vi "NIIE_MouseMove.vi"(7 "Buffer":refnum<queue>, 8 "Error":errorcluster, 9 "Coords":T5, 11 "Data":T1={"Class"={"Ants"=refnum, "Layer"=refnum, "Templates"=refnum, "Icon"=refnum, "Glyph"=refnum, "Settings"=refnum, "Tools"=refnum}, "Ref"={"Add Layer"=refnum, "Remove Layer"=refnum, "Line Text"=[], "Body Text Spec"=refnum, "DNL_Font"=refnum, "glyph path str"=refnum, "templates path str"=refnum, "Arrow Up"=refnum, "Arrow Down"=refnum, "IE VI Ref"=refnum, "Glyphs tree"=refnum, "Templates tree"=refnum, "Layer Icon Text"=refnum, "Layer Template"=refnum, "Clipboard"=refnum, "BW icon in"=refnum, "Color icon in"=refnum, "Layer Clust"=refnum, "Body Text"=refnum, "DNL_Framework Templates"=refnum, "Search Templates"=refnum, "TextMarker"=refnum, "Tab Control"=refnum, "Search Glyphs"=refnum, "Line Color"=refnum, "DNL_Glyphs []"=refnum, "Fill Color"=refnum, "Tools"=refnum, "Glyphs tree"=refnum, "Icon"=refnum, "Preview"=refnum, "Ants"=refnum, "Terminals"=refnum, "menu reference"=refnum, "LayerNames"=[], "GlyphLoadAnimation"=refnum, "TemplateLoadAnimation"=refnum, "refreshGlyphs"=refnum, "refreshTemplates"=refnum}, "Support"={"AntsRect"={"left"=0, "top"=0, "right"=0, "bottom"=0}, "Mouse Move Coords"={"Horizontal"=0, "Vertical"=0}, "Mouse Down Coords"={"Horizontal"=0, "Vertical"=0}, "Temp Coord"={"Horizontal"=0, "Vertical"=0}, "Action"=enum."Default", "Edge Color"=4914962, "Fill Color"=16860, "Mouse Down?"=FALSE, "Draft Mode?"=FALSE, "Temp Icon"=bytes[3102], "CTRL Pressed"=FALSE, "Move Selection?"=FALSE, "AntsRect Orig"={"left"=0, "top"=0, "right"=0, "bottom"=0}, "Text"="", "TM Set?"=FALSE, "Mouse inside icon?"=FALSE, "Tool (old value)"=0, "Pencil Move Color"=0, "Swap Colors?"=FALSE, "Shift pressed?"=FALSE}}) -> (0 "Error Out":errorcluster, 3 "Data Out":T1={"Class"={"Ants"=refnum, "Layer"=refnum, "Templates"=refnum, "Icon"=refnum, "Glyph"=refnum, "Settings"=refnum, "Tools"=refnum}, "Ref"={"Add Layer"=refnum, "Remove Layer"=refnum, "Line Text"=[], "Body Text Spec"=refnum, "DNL_Font"=refnum, "glyph path str"=refnum, "templates path str"=refnum, "Arrow Up"=refnum, "Arrow Down"=refnum, "IE VI Ref"=refnum, "Glyphs tree"=refnum, "Templates tree"=refnum, "Layer Icon Text"=refnum, "Layer Template"=refnum, "Clipboard"=refnum, "BW icon in"=refnum, "Color icon in"=refnum, "Layer Clust"=refnum, "Body Text"=refnum, "DNL_Framework Templates"=refnum, "Search Templates"=refnum, "TextMarker"=refnum, "Tab Control"=refnum, "Search Glyphs"=refnum, "Line Color"=refnum, "DNL_Glyphs []"=refnum, "Fill Color"=refnum, "Tools"=refnum, "Glyphs tree"=refnum, "Icon"=refnum, "Preview"=refnum, "Ants"=refnum, "Terminals"=refnum, "menu reference"=refnum, "LayerNames"=[], "GlyphLoadAnimation"=refnum, "TemplateLoadAnimation"=refnum, "refreshGlyphs"=refnum, "refreshTemplates"=refnum}, "Support"={"AntsRect"={"left"=0, "top"=0, "right"=0, "bottom"=0}, "Mouse Move Coords"={"Horizontal"=0, "Vertical"=0}, "Mouse Down Coords"={"Horizontal"=0, "Vertical"=0}, "Temp Coord"={"Horizontal"=0, "Vertical"=0}, "Action"=enum."Default", "Edge Color"=4914962, "Fill Color"=16860, "Mouse Down?"=FALSE, "Draft Mode?"=FALSE, "Temp Icon"=bytes[3102], "CTRL Pressed"=FALSE, "Move Selection?"=FALSE, "AntsRect Orig"={"left"=0, "top"=0, "right"=0, "bottom"=0}, "Text"="", "TM Set?"=FALSE, "Mouse inside icon?"=FALSE, "Tool (old value)"=0, "Pencil Move Color"=0, "Swap Colors?"=FALSE, "Shift pressed?"=FALSE}})   [LabVIEW 2021]
uses:
  <vilib>/Utility/miscctls.llb/LVPoint32TypeDef.ctl
  Controls/IE Data.ctl
  Class/Ants/Ants.lvclass
  Class/FakedArray/FakedArray.lvclass
  Class/Icon Library/Glyph.lvclass
  Class/Settings/Settings.lvclass
  Class/Tools/Tools Paint.lvclass
  vi.lib/LabVIEW Icon API/lv_icon/Classes/Icon/Icon.lvclass
  Controls/IE Classes.ctl
  Controls/References Cluster.ctl
  Controls/SupportClass.ctl
  Controls/ENUM_SupportClass_Action.ctl
  vi.lib/LabVIEW Icon API/lv_icon/Controls/IEColor.ctl
  vi.lib/LabVIEW Icon API/lv_icon/lv_icon.lvlib
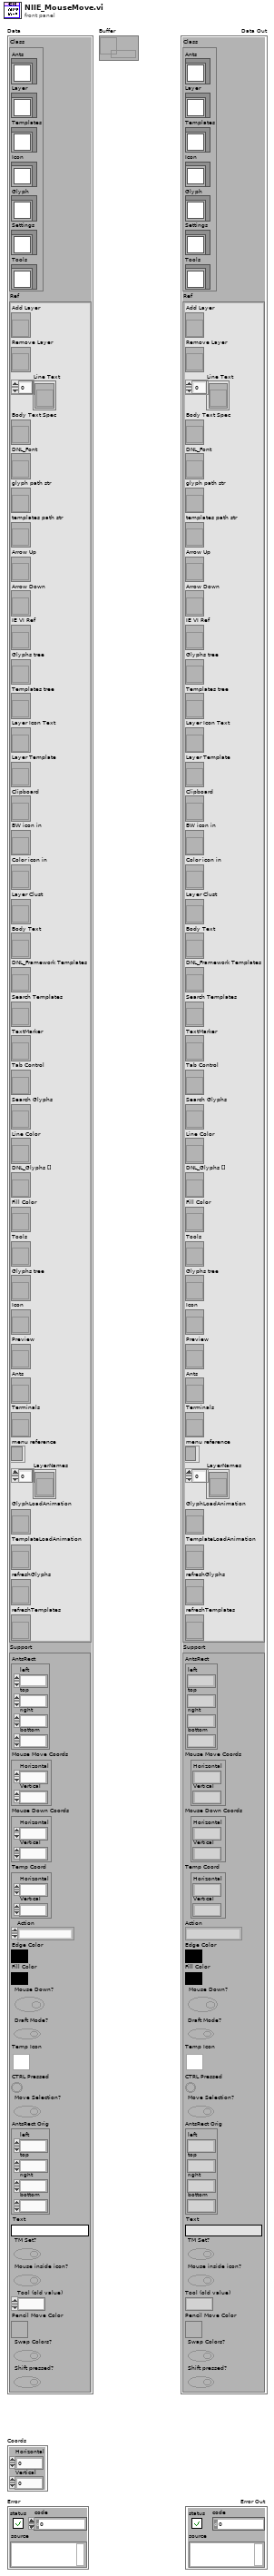
[diagram p1: front panel]
types:
  T1 = typedef "IE Data.ctl" = cluster{"Class":T2, "Ref":T3, "Support":T4}
  T2 = typedef "IE Classes.ctl" = cluster{"Ants":refnum<class "Ants.lvclass">, "Layer":refnum<class "FakedArray.lvclass">, "Templates":refnum<class "FakedArray.lvclass">, "Icon":refnum<class "Icon.lvclass">, "Glyph":refnum<class "Glyph.lvclass">, "Settings":refnum<class "Settings.lvclass">, "Tools":refnum<class "Tools Paint.lvclass">}
  T3 = typedef "References Cluster.ctl" = cluster{"Add Layer":refnum<vi>, "Remove Layer":refnum<vi>, "Line Text":refnum<vi>[], "Body Text Spec":refnum<vi>, "DNL_Font":refnum<vi>, "glyph path str":refnum<vi>, "templates path str":refnum<vi>, "Arrow Up":refnum<vi>, "Arrow Down":refnum<vi>, "IE VI Ref":refnum<vi>, "Glyphs tree":refnum<vi>, "Templates tree":refnum<vi>, "Layer Icon Text":refnum<vi>, "Layer Template":refnum<vi>, "Clipboard":refnum<vi>, "BW icon in":refnum<vi>, "Color icon in":refnum<vi>, "Layer Clust":refnum<vi>, "Body Text":refnum<vi>, "DNL_Framework Templates":refnum<vi>, "Search Templates":refnum<vi>, "TextMarker":refnum<vi>, "Tab Control":refnum<vi>, "Search Glyphs":refnum<vi>, "Line Color":refnum<vi>, "DNL_Glyphs []":refnum<vi>, "Fill Color":refnum<vi>, "Tools":refnum<vi>, "Glyphs tree":refnum<vi>, "Icon":refnum<vi>, "Preview":refnum<vi>, "Ants":refnum<vi>, "Terminals":refnum<vi>, "menu reference":refnum<k9>, "LayerNames":refnum<vi>[], "GlyphLoadAnimation":refnum<vi>, "TemplateLoadAnimation":refnum<vi>, "refreshGlyphs":refnum<vi>, "refreshTemplates":refnum<vi>}
  T4 = typedef "SupportClass.ctl" = cluster{"AntsRect":cluster{"left":i16, "top":i16, "right":i16, "bottom":i16}, "Mouse Move Coords":T5, "Mouse Down Coords":T5, "Temp Coord":T5, "Action":T6, "Edge Color":T7, "Fill Color":T7, "Mouse Down?":bool, "Draft Mode?":bool, "Temp Icon":picture, "CTRL Pressed":bool, "Move Selection?":bool, "AntsRect Orig":cluster{"left":i16, "top":i16, "right":i16, "bottom":i16}, "Text":string, "TM Set?":bool, "Mouse inside icon?":bool, "Tool (old value)":u32, "Pencil Move Color":u32, "Swap Colors?":bool, "Shift pressed?":bool}
  T5 = typedef "LVPoint32TypeDef.ctl" = cluster{"Horizontal":i32, "Vertical":i32}
  T6 = typedef "ENUM_SupportClass_Action.ctl" = enum16{"Default", "Move Selection", "Glyph Library", "Tool"}
  T7 = typedef "IEColor.ctl" = u32
  T8 = typedef "Cluster_Path&Icon.ctl" = cluster{"Rectangle":cluster{"left":i16, "top":i16, "right":i16, "bottom":i16}, "Path":path, "Image":picture, "Filter":string, "FileName":string}
  T9 = cluster{"left":i16, "top":i16, "right":i16, "bottom":i16}
  T10 = typedef "Cluster_Button Draw Tools.ctl" = enum32{"Pencil", "Line", "Dropper", "Fill", "Rectangle", "Filled Rectangle", "Ellipse", "Filled Ellipse", "Eraser", "Text", "Select", "Move"}
  T11 = cluster{"Horizontal":i32, "Vertical":i32, "Horizontal":i32, "Vertical":i32}
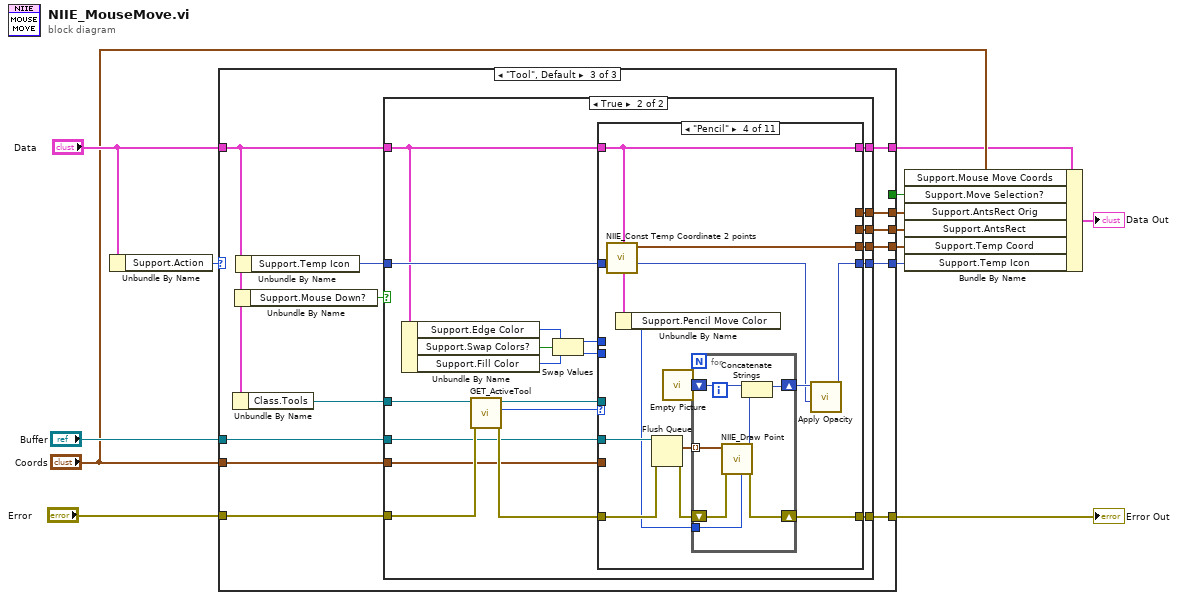
[diagram p0: block diagram]
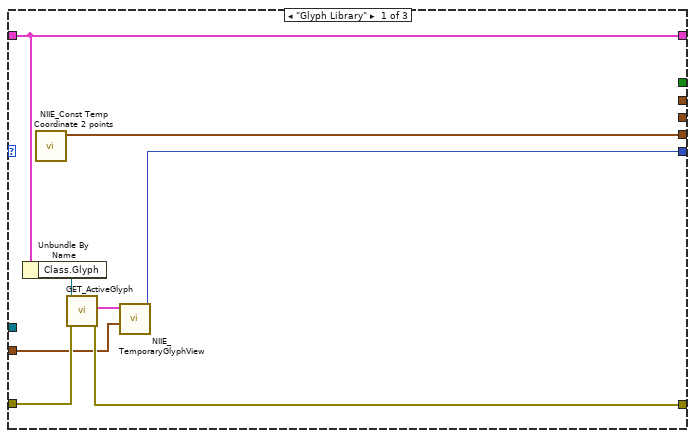
[diagram p2: hidden frame]
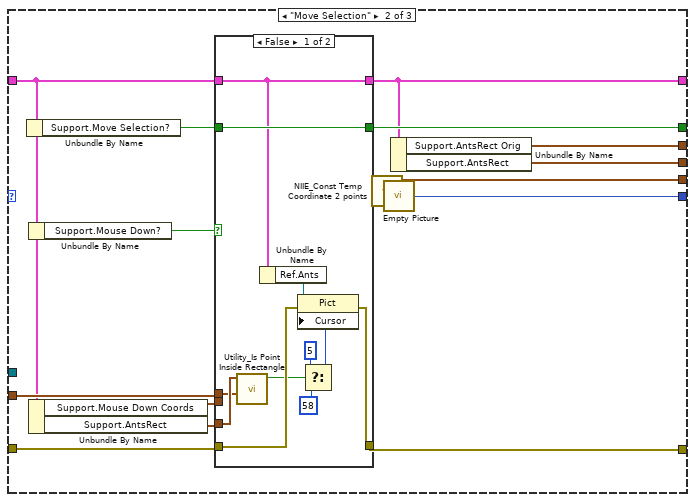
[diagram p3: hidden frame]
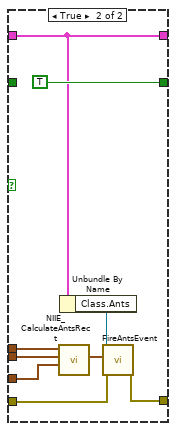
[diagram p4: hidden frame]
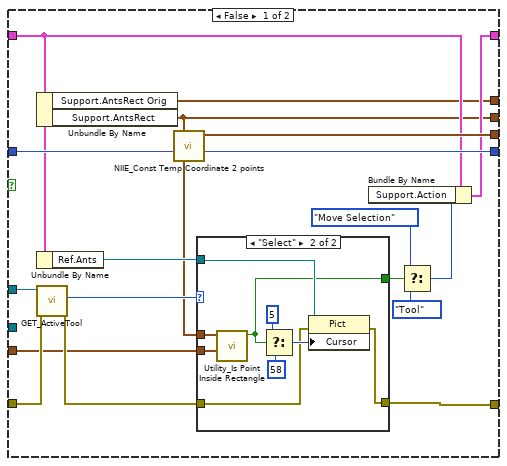
[diagram p5: hidden frame]
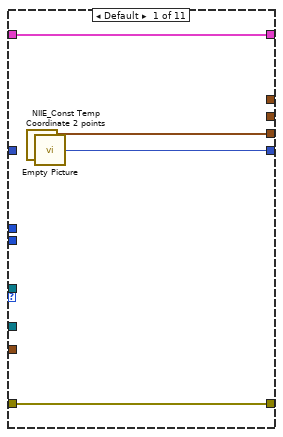
[diagram p7: hidden frame]
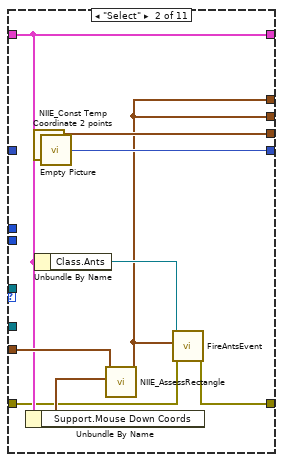
[diagram p8: hidden frame]
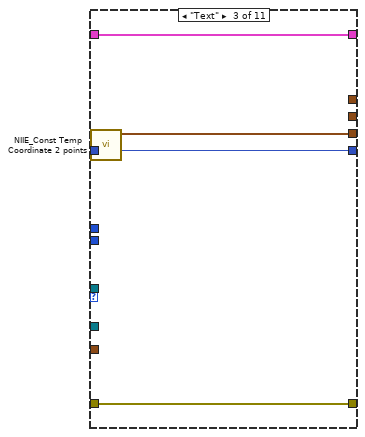
[diagram p9: hidden frame]
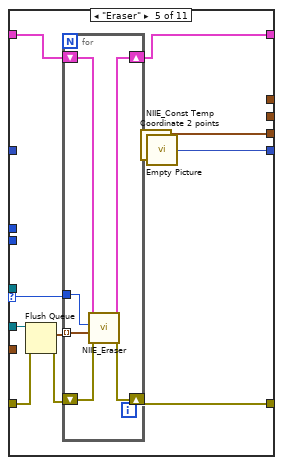
[diagram p10: hidden frame]
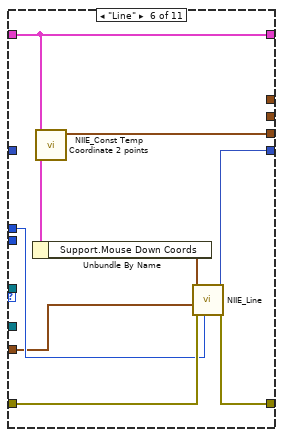
[diagram p11: hidden frame]
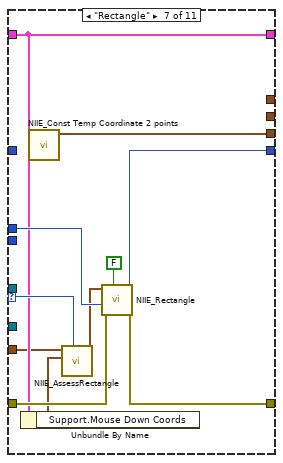
[diagram p12: hidden frame]
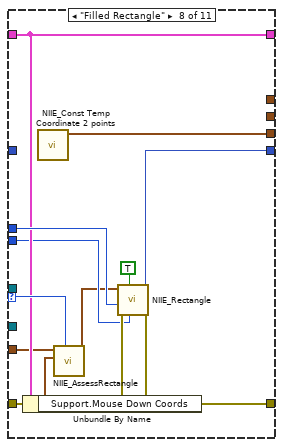
[diagram p13: hidden frame]
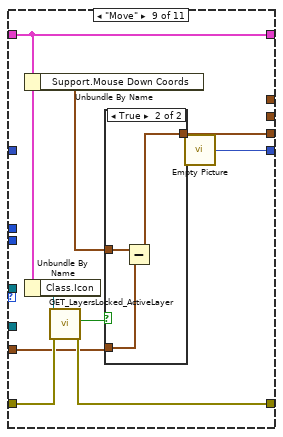
[diagram p14: hidden frame]
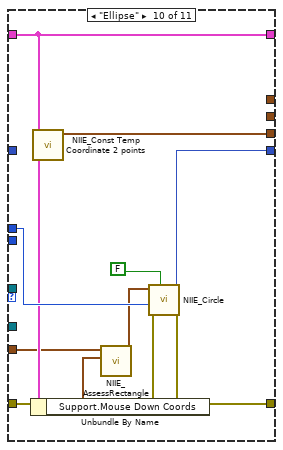
[diagram p16: hidden frame]
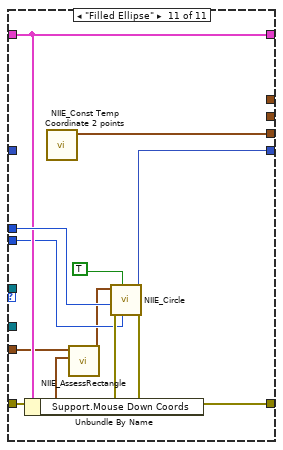
[diagram p17: hidden frame]
diagram:
  n1 = Unbundle By Name("Data") -> ("Support.Action"=w11:T6)
  n2 = case shown="\"Tool\", Default" w11 {
    tunnel: "Error" -> [w17 w33 w68]
    tunnel: [w20 w32 w67] -> w5
    tunnel: [w19 w34 w66] -> w12
    tunnel: [w18 w35 w65] -> w13
    tunnel: [_ w28 w64] -> w10
    tunnel: [_ w29 w63] -> w9
    tunnel: [_ w31 _] -> w8
    tunnel: "Buffer" -> [_ _ w62]
    tunnel: "Data" -> [w15 w23 w57]
    tunnel: [w15 w22 w61] -> w1
    tunnel: "Coords" -> [w14 w30 w60]
    frame "Glyph Library" {
      n3 = Unbundle By Name(w15) -> ("Class.Glyph"=w16:refnum<class "Glyph.lvclass">)
      n4 = call "NIIE_Const Temp Coordinate 2 points.vi"() -> ("Const Temp Coordinate"=w18:T5)  [unwired: 11 out]
      n5 = call-dynamic "GET_ActiveGlyph.vi"("Error"=w17, "Glyph.lvclass"=w16) -> ("Error Out"=w20:errorcluster, "Path And Icon Out"=w21:T8)  [unwired: 8 out]
      n6 = call "NIIE_TemporaryGlyphView.vi"("Mouse Coords Pic"=w14, "Path And Icon"=w21) -> ("Icon Out"=w19:picture)  [unwired: 9 out]
    }
    frame "Move Selection" {
      n7 = Unbundle By Name(w23) -> ("Support.Move Selection?"=w24:bool)
      n8 = Unbundle By Name(w23) -> ("Support.Mouse Down?"=w25:bool)
      n9 = Unbundle By Name(w23) -> ("Support.Mouse Down Coords"=w26:T5, "Support.AntsRect"=w27:T9)
      n10 = case shown="False" w25 {
        tunnel: w33 -> [w39 w55]
        tunnel: [w43 w54] -> w32
        tunnel: w30 -> [w40 w49]
        tunnel: w26 -> [_ w52]
        tunnel: w27 -> [w42 w51]
        tunnel: [w41 TRUE] -> w31
        tunnel: w24 -> [w41 _]
        tunnel: w23 -> [w37 w47]
        tunnel: [w37 w47] -> w22
        frame False {
          n11 = call "Utility_Is Point Inside Rectangle.vi"("Point"=w40, "Rectangle"=w42) -> ("Inside? Out"=w36:bool)  [unwired: 9 out]
          n12 = Unbundle By Name(w37) -> ("Ref.Ants"=w38:refnum<vi>)
          n13 = Select(t=5 ("Cursor"), s=w36, f=58 ("Cursor")) -> (s? t:f=w44:i32)
          n14 = property class="Pict"(reference=w38, error in=w39, "Cursor"=w44) -> (error out=w43:errorcluster)  [unwired: 1 out]
        }
        frame True {
          n15 = call "NIIE_CalculateAntsRect.vi"("AntsRect"=w51, "Mouse Down Coords"=w52, "Mouse Move Coords"=w49) -> ("Rect"=w50:cluster{i32, i32, i32, i32})  [unwired: 8 out]
          n16 = Unbundle By Name(w47) -> ("Class.Ants"=w48:refnum<class "Ants.lvclass">)
          n17 = call "FireAntsEvent.vi"("error in (no error)"=w55, "Rectangle (default: deselect)"=w50, "Ants in"=w48) -> ("error out"=w54:errorcluster)  [unwired: 1 in, 7 out]
        }
      }
      n18 = call "NIIE_Const Temp Coordinate 2 points.vi"() -> ("Const Temp Coordinate"=w35:T5)  [unwired: 11 out]
      n19 = call "Empty Picture"() -> ("empty picture"=w34:picture)
      n20 = Unbundle By Name(w22) -> ("Support.AntsRect Orig"=w29:T9, "Support.AntsRect"=w28:T9)
    }
    frame "Tool", Default {
      n21 = Unbundle By Name(w57) -> ("Class.Tools"=w59:refnum<class "Tools Paint.lvclass">)
      n22 = Unbundle By Name(w57) -> ("Support.Mouse Down?"=w58:bool)
      n23 = Unbundle By Name(w57) -> ("Support.Temp Icon"=w56:picture)
      n24 = case shown="True" w58 {
        tunnel: w68 -> [w78 w115]
        tunnel: w56 -> [w77 w112]
        tunnel: [w82 w110] -> w67
        tunnel: [w77 w109] -> w66
        tunnel: [w85 w108] -> w65
        tunnel: [w70 w107] -> w64
        tunnel: [w69 w106] -> w63
        tunnel: w59 -> [w79 w105]
        tunnel: w62 -> [_ w104]
        tunnel: w57 -> [w72 w98]
        tunnel: [w76 w103] -> w61
        tunnel: w60 -> [w73 w102]
        frame False {
          n25 = Unbundle By Name(w72) -> ("Support.AntsRect Orig"=w69:T9, "Support.AntsRect"=w70:T9)
          n26 = Unbundle By Name(w72) -> ("Ref.Ants"=w74:refnum<vi>)
          n27 = call-dynamic "GET_ActiveTool.vi"("error in (no error)"=w78, "Tools Paint.lvclass in"=w79) -> ("error out"=w84:errorcluster, "Radio Buttons"=w83:T10)  [unwired: 8 out]
          n28 = call "NIIE_Const Temp Coordinate 2 points.vi"() -> ("Const Temp Coordinate"=w85:T5)  [unwired: 11 out]
          n29 = case shown="\"Select\"" w83 {
            tunnel: w84 -> [w86 w89]
            tunnel: w73 -> [_ w92]
            tunnel: [w86 w91] -> w82
            tunnel: w70 -> [_ w90]
            tunnel: [_ w87] -> w81
            tunnel: w74 -> [_ w88]
            frame Default {
            }
            frame "Select" {
              n30 = call "Utility_Is Point Inside Rectangle.vi"("Point"=w92, "Rectangle"=w90) -> ("Inside? Out"=w87:bool)  [unwired: 9 out]
              n31 = Select(t=5 ("Cursor"), s=w87, f=58 ("Cursor")) -> (s? t:f=w93:i32)
              n32 = property class="Pict"(reference=w88, error in=w89, "Cursor"=w93) -> (error out=w91:errorcluster)  [unwired: 1 out]
            }
          }
          n33 = Select(t=ENUM_SupportClass_Action."Move Selection", s=w81, f=ENUM_SupportClass_Action."Tool" ("t")) -> (s? t:f=w75:T6)
          n34 = Bundle By Name(cluster=w72, "Support.Action"=w75) -> (w76:T1)
        }
        frame True {
          n35 = Unbundle By Name(w98) -> ("Support.Edge Color"=w100:T7, "Support.Swap Colors?"=w101:bool, "Support.Fill Color"=w99:T7)
          n36 = call-dynamic "GET_ActiveTool.vi"("error in (no error)"=w115, "Tools Paint.lvclass in"=w105) -> ("error out"=w113:errorcluster, "Radio Buttons"=w114:T10, "Tools Paint.lvclass out"=w111:refnum<class "Tools Paint.lvclass">)  [unwired: 7 out]
          n37 = Swap Values(12:w100, 13:w101, 14:w99) -> (1:w96:T7, 3:w97:T7)
          n38 = case shown="\"Pencil\"" w114 {
            selector: w114 -> [_ _ _ _ w159 _ w183 w195 _ _ _]
            tunnel: w113 -> [w119 w120 w132 w136 w154 w175 w186 w198 w204 w220 w231]
            tunnel: w112 -> [_ _ w131 w137 _ _ _ _ _ _ _]
            tunnel: w111 -> [_ _ _ _ _ _ _ _ _ _ _]
            tunnel: w96 -> [_ _ _ _ _ w173 w184 w196 _ w218 w229]
            tunnel: [w119 w121 w132 w144 w161 w174 w185 w197 w206 w219 w230] -> w110
            tunnel: [w118 w127 w131 w143 w160 w168 w176 w187 w207 w212 w222] -> w109
            tunnel: [w117 w128 w130 w142 w158 w172 w182 w194 w201 w217 w228] -> w108
            tunnel: [_ w122 _ _ _ _ _ _ _ _ _] -> w107
            tunnel: [_ w122 _ _ _ _ _ _ _ _ _] -> w106
            tunnel: w97 -> [_ _ _ _ _ _ _ w191 _ _ w224]
            tunnel: w104 -> [_ _ _ w141 w155 _ _ _ _ _ _]
            tunnel: w98 -> [w116 w124 w129 w134 w157 w171 w181 w193 w200 w215 w226]
            tunnel: [w116 w124 w129 w134 w156 w171 w181 w193 w200 w215 w226] -> w103
            tunnel: w102 -> [_ w125 _ _ _ w170 w178 w189 w199 w213 w223]
            frame Default {
              n39 = call "NIIE_Const Temp Coordinate 2 points.vi"() -> ("Const Temp Coordinate"=w117:T5)  [unwired: 11 out]
              n40 = call "Empty Picture"() -> ("empty picture"=w118:picture)
            }
            frame "Select" {
              n41 = Unbundle By Name(w124) -> ("Support.Mouse Down Coords"=w126:T5)
              n42 = call "NIIE_Const Temp Coordinate 2 points.vi"() -> ("Const Temp Coordinate"=w128:T5)  [unwired: 11 out]
              n43 = Unbundle By Name(w124) -> ("Class.Ants"=w123:refnum<class "Ants.lvclass">)
              n44 = call "Empty Picture"() -> ("empty picture"=w127:picture)
              n45 = call "NIIE_AssessRectangle.vi"(10:"Coords"=w126, 11:"Coords"=w125) -> ("Rectangle Out"=w122:T11)  [unwired: 9 in]
              n46 = call "FireAntsEvent.vi"("error in (no error)"=w120, "Rectangle (default: deselect)"=w122, "Ants in"=w123) -> ("error out"=w121:errorcluster)  [unwired: 1 in, 7 out]
            }
            frame "Text" {
              n47 = call "NIIE_Const Temp Coordinate 2 points.vi"() -> ("Const Temp Coordinate"=w130:T5)  [unwired: 11 out]
            }
            frame "Pencil" {
              n48 = call "NIIE_Const Temp Coordinate 2 points.vi"() -> ("Const Temp Coordinate"=w142:T5)  [unwired: 11 out]
              n49 = Unbundle By Name(w134) -> ("Support.Pencil Move Color"=w133:u32)
              n50 = Flush Queue(queue=w141, error in (no error)=w136) -> (remaining elements=w135:T5[], error out=w140:errorcluster)  [unwired: 1 out]
              n51 = call "Empty Picture"() -> ("empty picture"=w139:picture)
              n52 = for {
                shift-right: [w151] -> w144
                shift-left: w140 -> [w150]
                tunnel: w135 -> [w145] mode=indexing
                shift-right: [w148] -> w138
                shift-left: w139 -> [w149]
                tunnel: w133 -> [w147]
                n53 = call "NIIE_Draw Point.vi"("Edge Color"=w147, "Error"=w150, "Point(x,y)"=w145) -> ("Error Out"=w151:errorcluster, "New Picture Out"=w146:picture)  [unwired: 6 in, 1 out]
                n54 = Concatenate Strings(w149, w146) -> (w148:picture)
              }
              n55 = call "Apply Opacity.vi"("Bottom"=w137, "Top"=w138) -> ("new picture"=w143:picture)  [unwired: 1 in, 8 out]
            }
            frame "Eraser" {
              n56 = Flush Queue(queue=w155, error in (no error)=w154) -> (remaining elements=w152:T5[], error out=w153:errorcluster)  [unwired: 1 out]
              n57 = for {
                tunnel: w159 -> [w165]
                shift-right: [w163] -> w156
                shift-left: w157 -> [w164]
                tunnel: w152 -> [w162] mode=indexing
                shift-right: [w167] -> w161
                shift-left: w153 -> [w166]
                n58 = call "NIIE_Eraser.vi"("Error"=w166, "Point Out"=w162, "Radio Buttons"=w165, "Data"=w164) -> ("Error Out"=w167:errorcluster, "Data Out"=w163:T1)  [unwired: 6 out]
              }
              n59 = call "NIIE_Const Temp Coordinate 2 points.vi"() -> ("Const Temp Coordinate"=w158:T5)  [unwired: 11 out]
              n60 = call "Empty Picture"() -> ("empty picture"=w160:picture)
            }
            frame "Line" {
              n61 = Unbundle By Name(w171) -> ("Support.Mouse Down Coords"=w169:T5)
              n62 = call "NIIE_Const Temp Coordinate 2 points.vi"() -> ("Const Temp Coordinate"=w172:T5)  [unwired: 11 out]
              n63 = call "NIIE_Line.vi"("Color(black)"=w173, "Error"=w175, "End Point"=w170, "New Position"=w169) -> ("Error Out"=w174:errorcluster, "New Picture Out"=w168:picture)  [unwired: 6 in]
            }
            frame "Rectangle" {
              n64 = Unbundle By Name(w181) -> ("Support.Mouse Down Coords"=w180:T5)
              n65 = call "NIIE_Const Temp Coordinate 2 points.vi"() -> ("Const Temp Coordinate"=w182:T5)  [unwired: 11 out]
              n66 = call "NIIE_AssessRectangle.vi"("Tool"=w183, 10:"Coords"=w180, 11:"Coords"=w178) -> ("Rectangle Out"=w177:T11)  [unwired: 8 in]
              n67 = call "NIIE_Rectangle.vi"("Fill?(F)"=FALSE, "Error"=w186, "Edge Color"=w184, "Rect"=w177) -> ("Error Out"=w185:errorcluster, "New Picture Out"=w176:picture)  [unwired: 6 in]
            }
            frame "Filled Rectangle" {
              n68 = Unbundle By Name(w193) -> ("Support.Mouse Down Coords"=w192:T5)
              n69 = call "NIIE_Const Temp Coordinate 2 points.vi"() -> ("Const Temp Coordinate"=w194:T5)  [unwired: 11 out]
              n70 = call "NIIE_AssessRectangle.vi"("Tool"=w195, 10:"Coords"=w192, 11:"Coords"=w189) -> ("Rectangle Out"=w188:T11)  [unwired: 8 in]
              n71 = call "NIIE_Rectangle.vi"("Fill Color"=w191, "Fill?(F)"=TRUE, "Error"=w198, "Edge Color"=w196, "Rect"=w188) -> ("Error Out"=w197:errorcluster, "New Picture Out"=w187:picture)  [unwired: 5 in]
            }
            frame "Move" {
              n72 = Unbundle By Name(w200) -> ("Support.Mouse Down Coords"=w202:T5)
              n73 = Unbundle By Name(w200) -> ("Class.Icon"=w203:refnum<class "Icon.lvclass">)
              n74 = call-dynamic "GET_LayersLocked_ActiveLayer.vi"("error in (no error)"=w204, "Icon.lvclass in"=w203) -> ("error out"=w206:errorcluster, "Layers Locked?"=w205:bool)  [unwired: 8 out]
              n75 = case shown="True" w205 {
                tunnel: w202 -> [_ w210]
                tunnel: [_ w209] -> w201
                tunnel: w199 -> [_ w208]
                frame False {
                }
                frame True {
                  n76 = Subtract(x=w210, y=w208) -> (x-y=w209:T5)
                }
              }
              n77 = call "Empty Picture"() -> ("empty picture"=w207:picture)
            }
            frame "Ellipse" {
              n78 = Unbundle By Name(w215) -> ("Support.Mouse Down Coords"=w214:T5)
              n79 = call "NIIE_Const Temp Coordinate 2 points.vi"() -> ("Const Temp Coordinate"=w217:T5)  [unwired: 11 out]
              n80 = call "NIIE_AssessRectangle.vi"(10:"Coords"=w214, 11:"Coords"=w213) -> ("Rectangle Out"=w211:T11)  [unwired: 9 in]
              n81 = call "NIIE_Circle.vi"("Fill?(F)"=FALSE, "Error"=w220, "Edge Color"=w218, "Rect"=w211) -> ("Error Out"=w219:errorcluster, "New Picture Out"=w212:picture)  [unwired: 6 in]
            }
            frame "Filled Ellipse" {
              n82 = Unbundle By Name(w226) -> ("Support.Mouse Down Coords"=w225:T5)
              n83 = call "NIIE_Const Temp Coordinate 2 points.vi"() -> ("Const Temp Coordinate"=w228:T5)  [unwired: 11 out]
              n84 = call "NIIE_AssessRectangle.vi"(10:"Coords"=w225, 11:"Coords"=w223) -> ("Rectangle Out"=w221:T11)  [unwired: 9 in]
              n85 = call "NIIE_Circle.vi"("Fill Color"=w224, "Fill?(F)"=TRUE, "Error"=w231, "Edge Color"=w229, "Rect"=w221) -> ("Error Out"=w230:errorcluster, "New Picture Out"=w222:picture)  [unwired: 5 in]
            }
          }
        }
      }
    }
  }
  "Error Out" <- w5
  n86 = Bundle By Name(cluster=w1, "Support.Mouse Move Coords"="Coords", "Support.Move Selection?"=w8, "Support.AntsRect Orig"=w9, "Support.AntsRect"=w10, "Support.Temp Coord"=w13, "Support.Temp Icon"=w12) -> (→"Data Out":T1)
